vi "Construct.vi"(8 "error in (no error)":errorcluster, 11 "id":string) -> (0 "error out":errorcluster, 3 "Execution Unit Implementation":refnum<class "Execution Unit Implementation.lvclass">)   [LabVIEW 2020, in "Communication Bus Template Engine.lvlib" / "Implementation.lvlib" / "Execution Unit Implementation.lvclass"]
uses:
  Execution Unit Implementation.lvclass
  Execution Unit Implementation.lvclass/Execution Unit Implementation.ctl
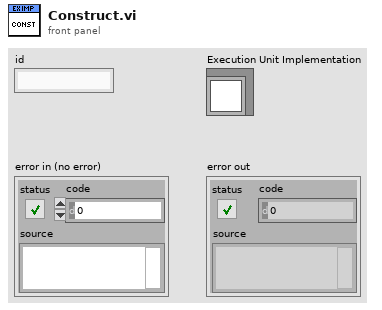
[diagram p1: front panel]
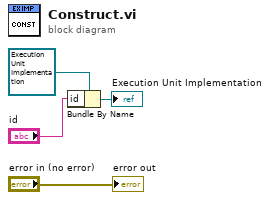
[diagram p0: block diagram]
diagram:
  n1 = Bundle By Name(cluster=refnum<class "Execution Unit Implementation.lvclass"> refnum ("Execution Unit Implementation"), "id"="id") -> (→"Execution Unit Implementation":refnum<class "Execution Unit Implementation.lvclass">)
  "error out" <- "error in (no error)"
